vi "AudioTest.SoundCheck Data Log Analysis_Module.vi"(6 "PlotColors":u32[](array[colorbox])=[56063, 16776722, 16730898, 16711925, 6618880], 7 "LimColors":u32[](array[colorbox])=[16448250, 16448250, 16448250, 16448250, 16448250, 16448250], 11 "Module Config":T3={"Name"="AudioGraphs", "Parent Q"=refnum, "Is Child?"=FALSE, "Index"=0, "Dirs"={"Root"=path "", "Config"=path "C:/MTE/Audio Test/Config", "Logs"=path "", "Reports"=path "", "App Data"=path ""}, "Simulate"=FALSE, "SimCtrl"=refnum}) -> ()   [LabVIEW 2018]
uses:
  <vilib>/KATE/Module/Module Config.ctl
  <vilib>/KATE/Queues/Q.Element.ctl
  <vilib>/KATE/Module/Module.Working Dirs.ctl
  Common/Utils/Results/Result.Measurement Item.ctl
  Common/Utils/Results/Result.Measurement and Attribute Item Status.ctl
  TypeDefs/AudioTest.Analysis Data Record.ctl
  Common/Utils/Errors/Error.Error Code List.ctl
  <vilib>/KATE/Queues/Queue Utils.lvlib
  <vilib>/KATE/Files/File Utils.lvlib
  <vilib>/KATE/Time/Time Utils.lvlib
  <vilib>/KATE/Module/Module Utils.lvlib
panel:
  in  "Main Tab":enum32{"Graphs", "Results", "Setup"}(tab)
  in  "Graph - Open Composite":bool
  in  "Go To Results":bool
  in  "Graph Wins - Reset Pos":bool
  in  "Graph Wins - Close":bool
  in  "Graph Wins - Open":bool
  in  "Save to CSV":bool
  in  "X Scale":enum16{"Log", "Linear"}(ring)
  out "Y Units":string
  out "X Units":string
  in  "Next":bool
  in  "Prev":bool
  out "XY Graph":cluster{"X":dbl[], "Y":dbl[]}[](graph)
  in  "Plot":u16(ring)
  in  "SoundCheck Data File":path caption="Data File"
  in  "Load File":bool
  in  "Go To Setup":bool
  in  "Go To Graphs":bool
  out "Meas Data":T1[](array[typedef]) {"Status" items=["LOG", "PASS", "FAIL", "ERROR"]}
  in  "Reinit Config":bool
  out "Graph Cnt":i32
  out "Error":errorcluster
  out "Q Name":string="AudioGraphs"
  in  "Go To Graphs 2":bool
  # "Indiv Graphs"
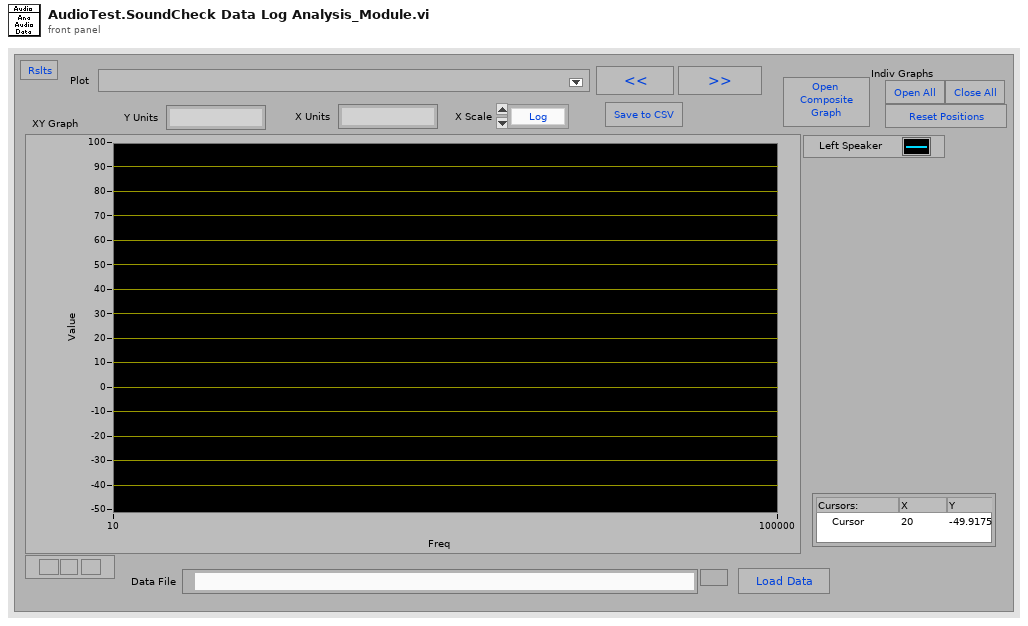
[diagram p1: front panel]
types:
  T1 = typedef "Result.Measurement Item.ctl" = cluster{"Cnt":i32, "Step":string, "Category":string, "Name":string, "Value":string, "Units":string, "LimType":string, "LL":string, "UL":string, "Status":T2, "Code":i32, "Desc":string, "Time":timestamp}
  T2 = typedef "Result.Measurement and Attribute Item Status.ctl" = i32
  T3 = typedef "KATE_Lib.lvlib/Module Utils.lvlib/Module Config.ctl" = cluster{"Name":string, "Parent Q":refnum<queue>, "Is Child?":bool, "Index":i32, "Dirs":T4, "Simulate":bool, "SimCtrl":refnum<vi>}
  T4 = typedef "KATE_Lib.lvlib/Module Utils.lvlib/Module.Working Dirs.ctl" = cluster{"Root":path, "Config":path, "Logs":path, "Reports":path, "App Data":path}
  T5 = typedef "AudioTest.Analysis Data Record.ctl" = cluster{"Name":string, "X Units":string, "Y Units":string, "DataPlots":cluster{"X":dbl[], "Y":dbl[]}[], "LimitPlots":cluster{"X":dbl[], "Y":dbl[]}[], "DataPlotNames":string[], "LimitPlotNames":string[], "Fail":bool}
  T6 = enum32{"invalid app kind", "Development System", "Run Time System", "Student Edition", "Embedded LabVIEW", "Evaluation", "Custom"}
  T7 = cluster{"Graphs":T5[], "Config Dir":path, "PlotColors":u32[], "LimColors":u32[], "PlotWins":cluster{"Name":string, "vi ref":refnum<vi>}[], "PlotComp":cluster{"Name":string, "vi ref":refnum<vi>}}
  T8 = typedef "Error.Error Code List.ctl" = i32
  T9 = typedef "KATE_Lib.lvlib/Queue Utils.lvlib/Q.Element.ctl" = cluster{"Cmd":string, "Sub":string, "Data1":variant, "Data2":variant}
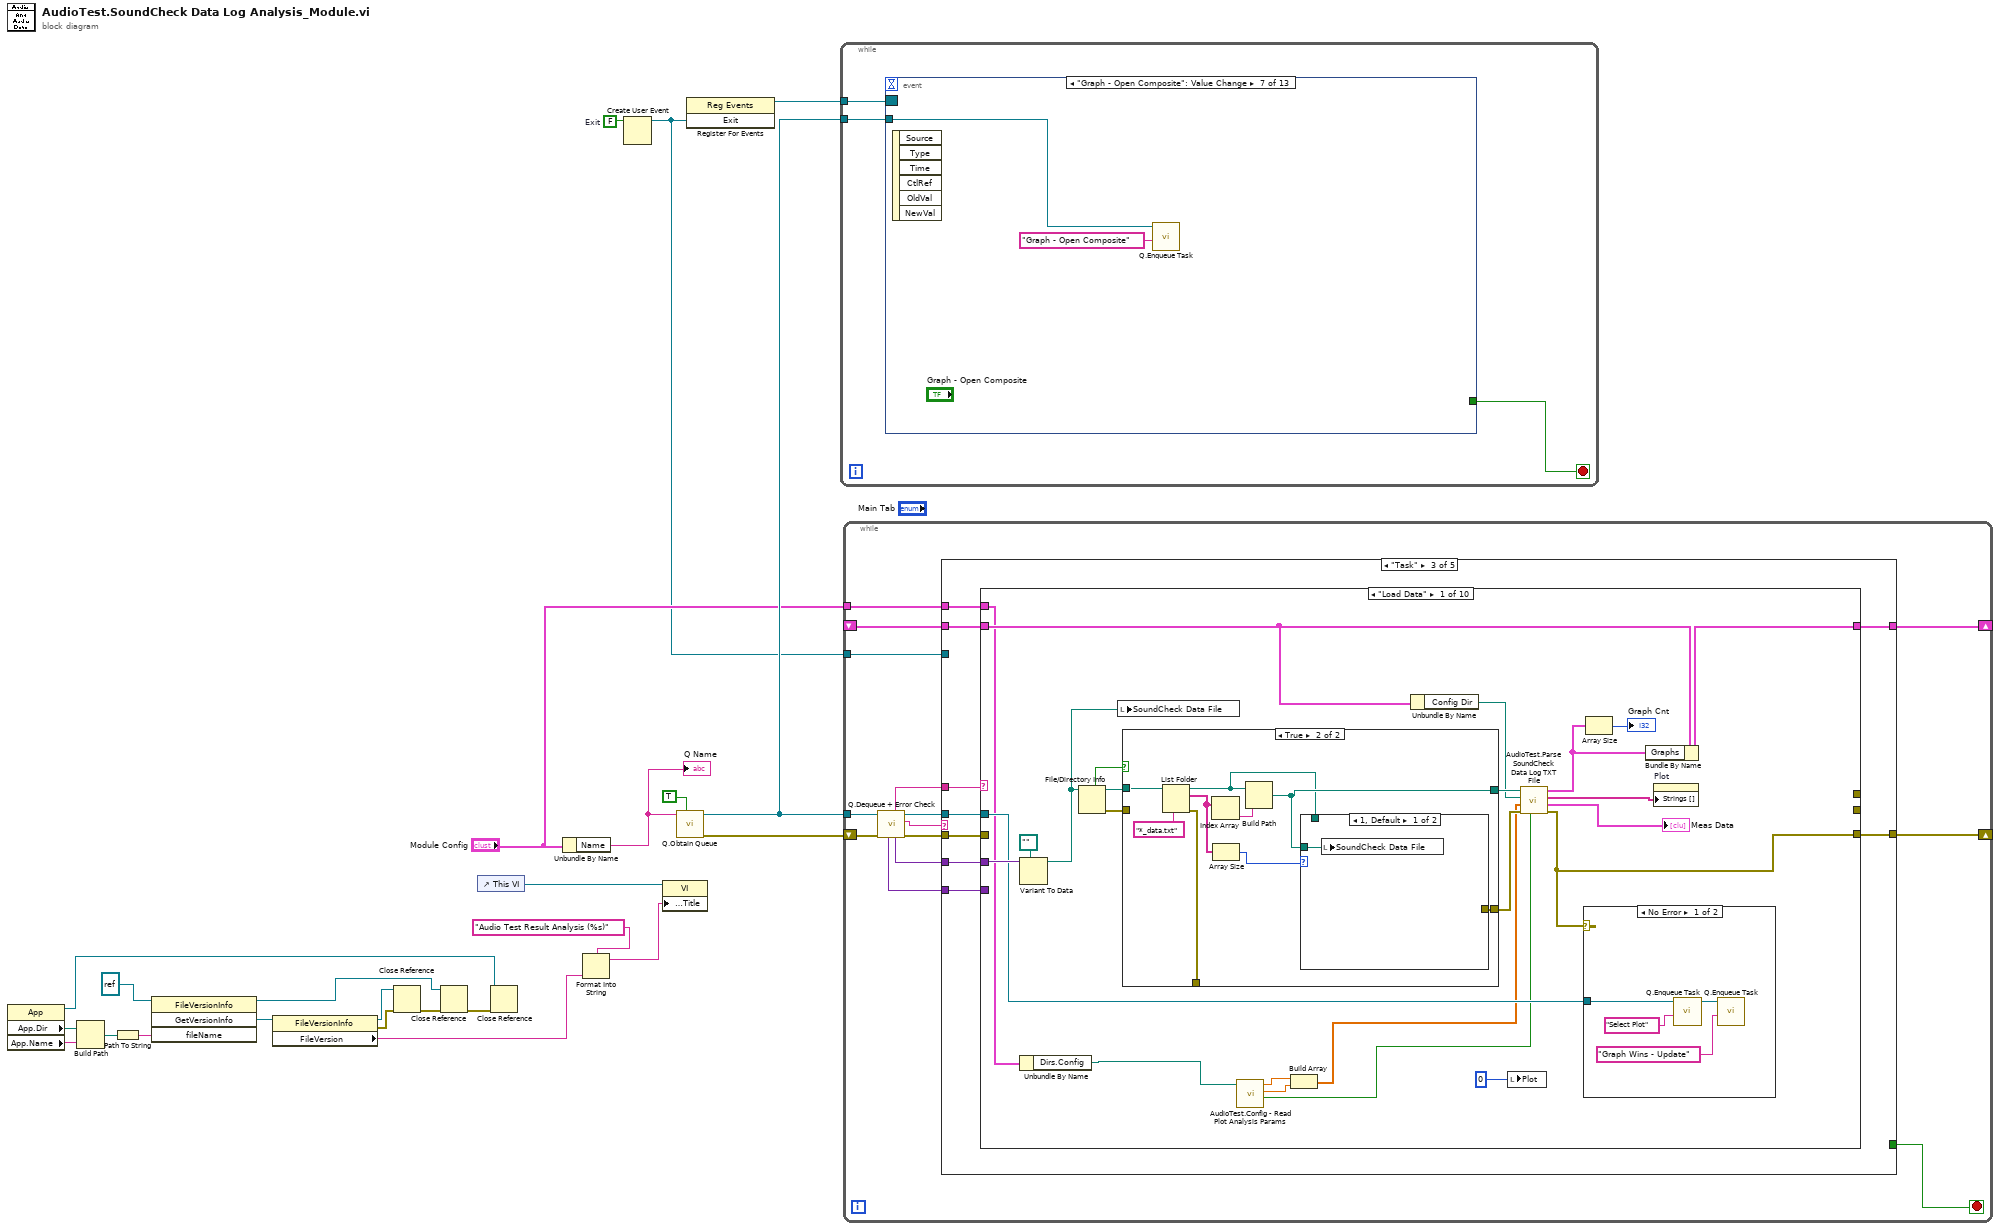
[diagram p0: block diagram]
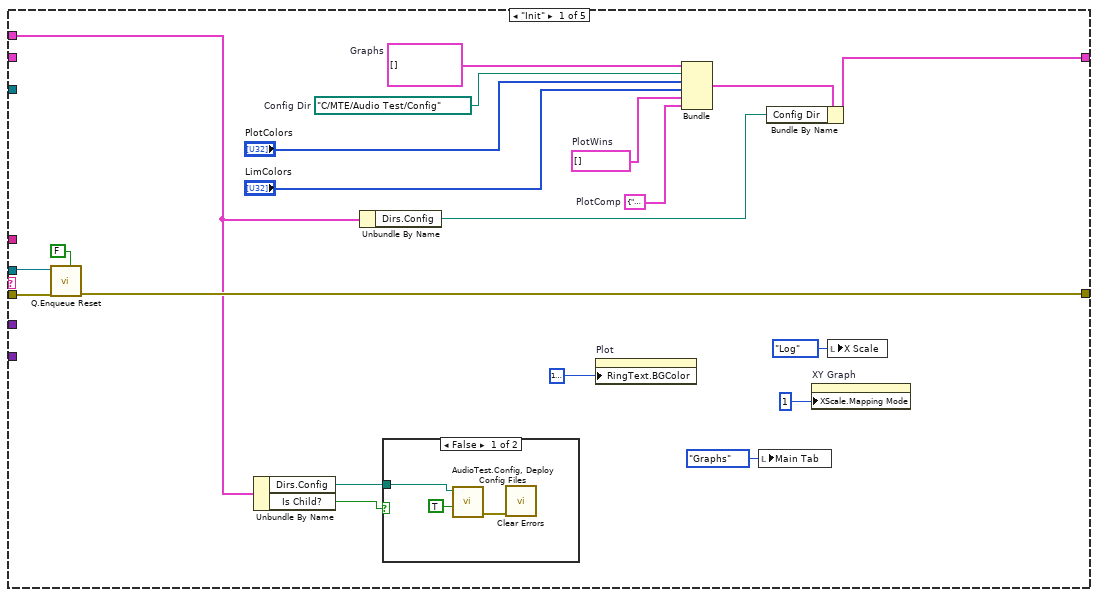
[diagram p2: hidden frame]
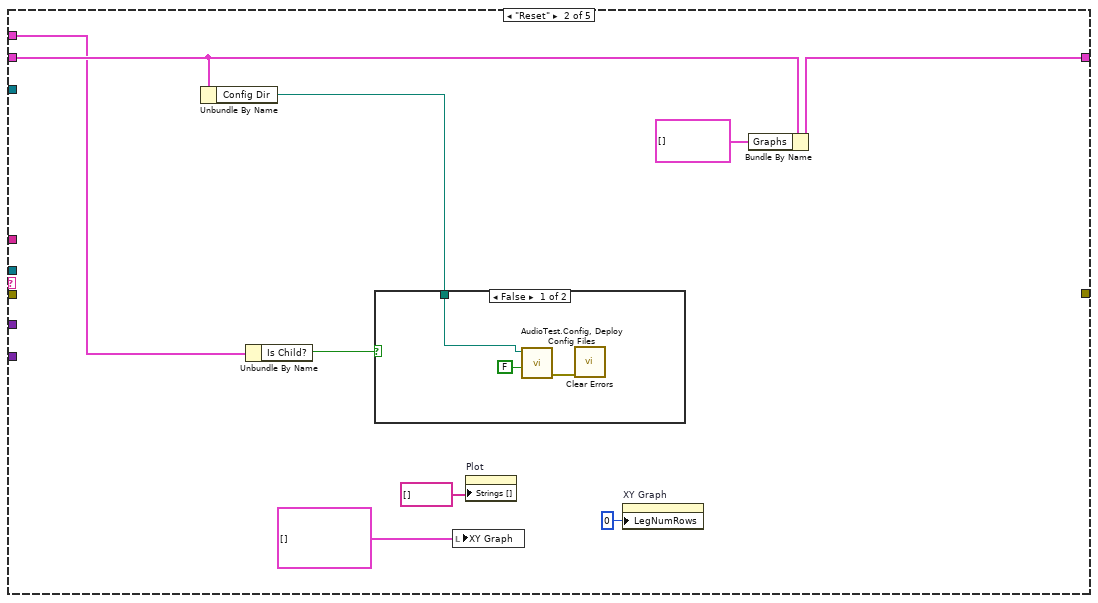
[diagram p4: hidden frame]
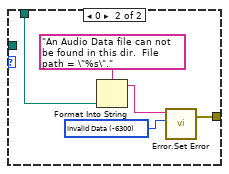
[diagram p8: hidden frame]
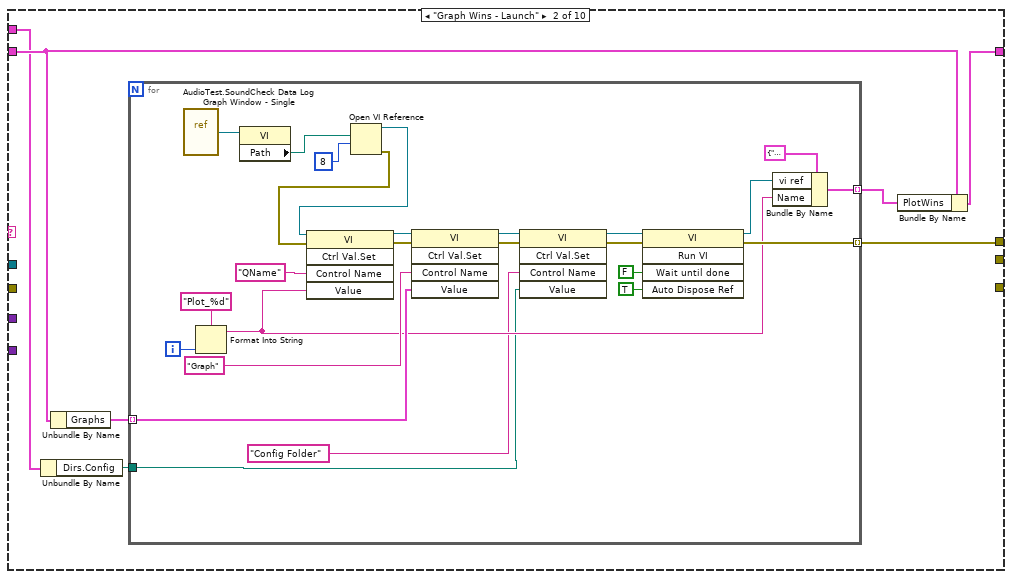
[diagram p9: hidden frame]
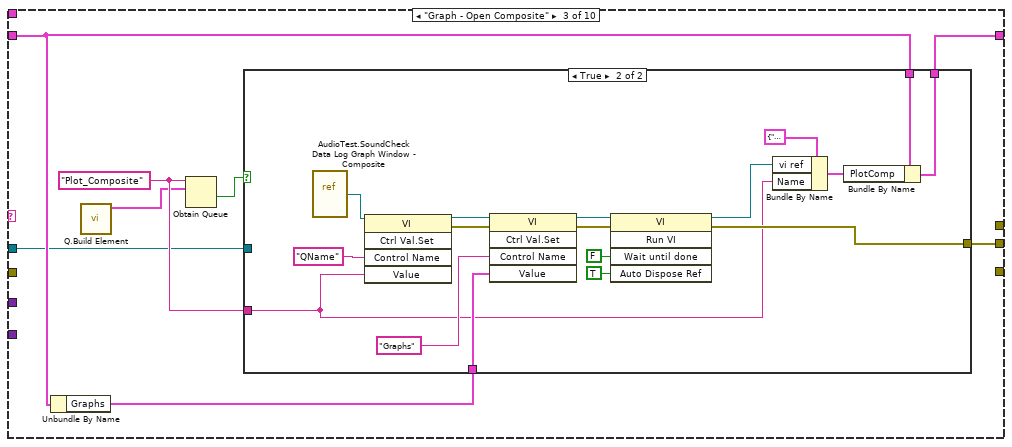
[diagram p10: hidden frame]
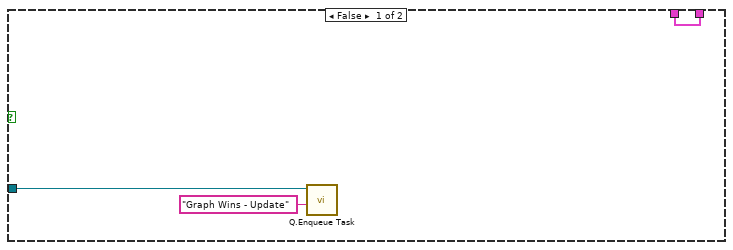
[diagram p11: hidden frame]
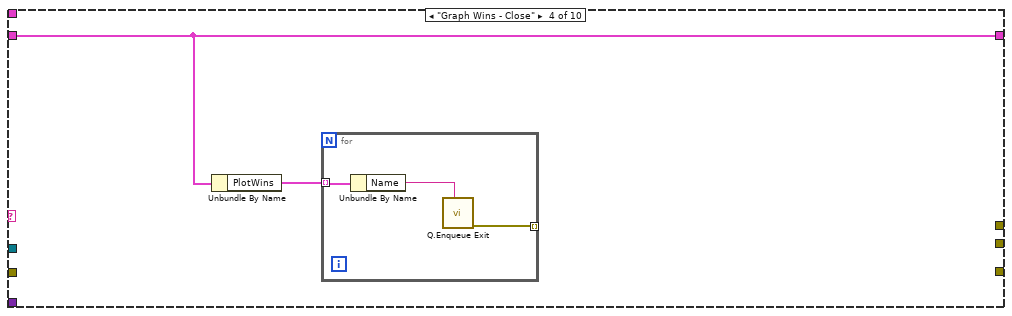
[diagram p12: hidden frame]
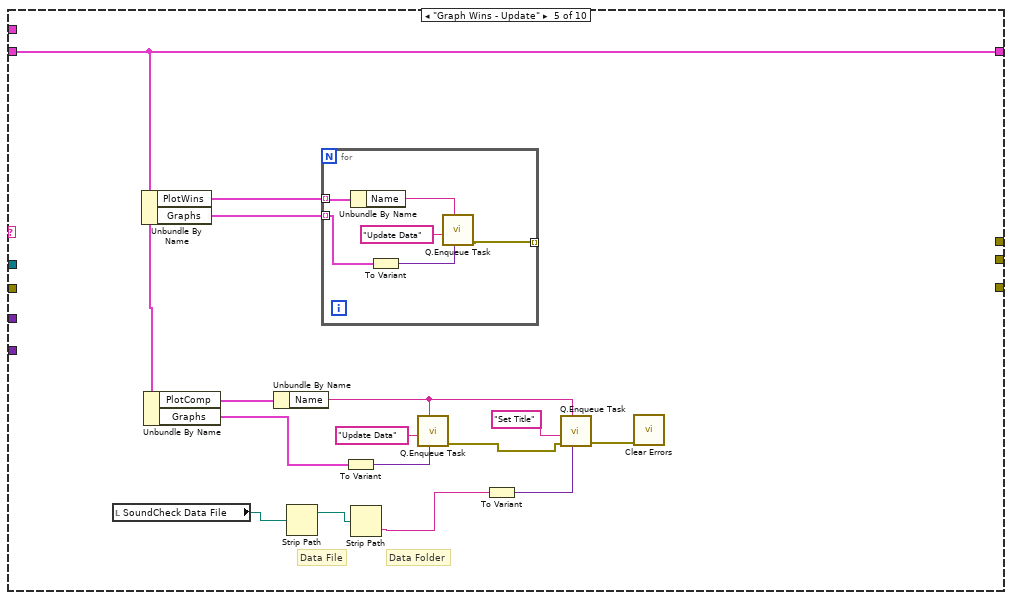
[diagram p13: hidden frame]
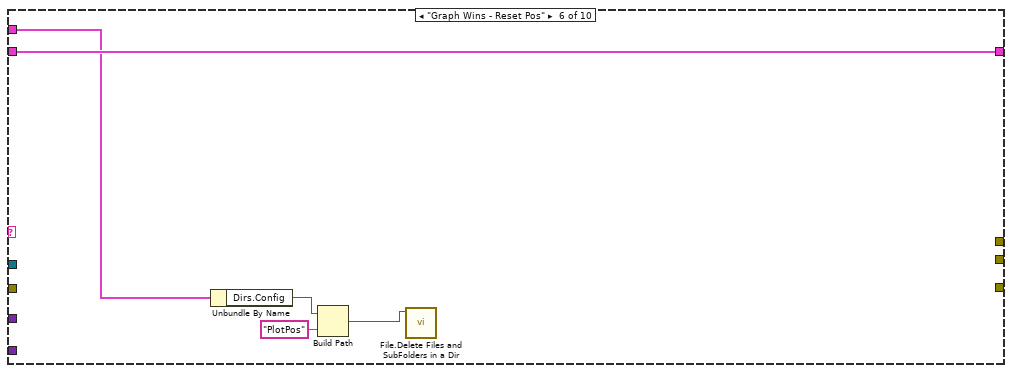
[diagram p14: hidden frame]
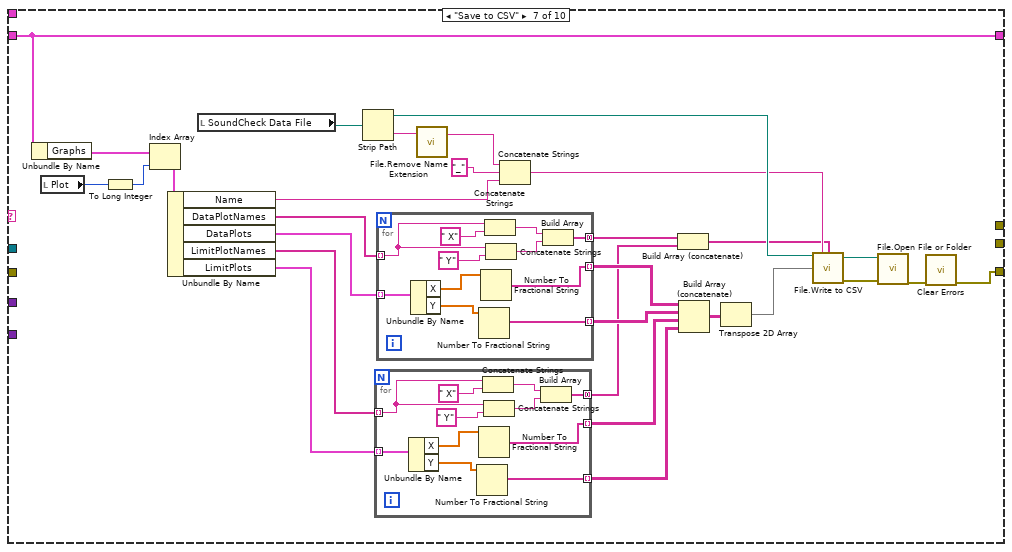
[diagram p15: hidden frame]
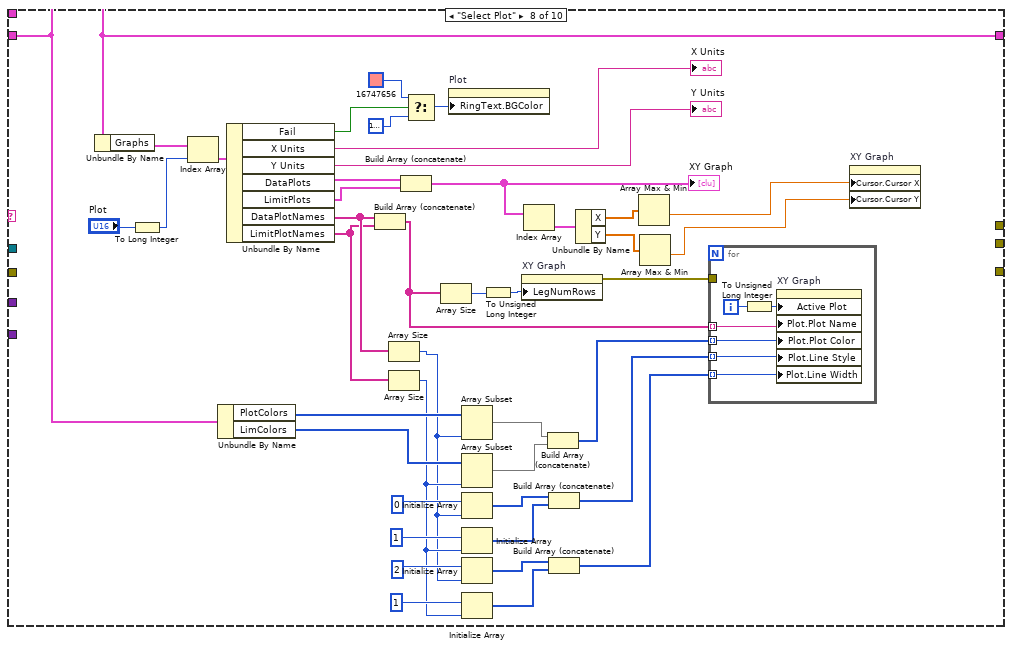
[diagram p16: hidden frame]
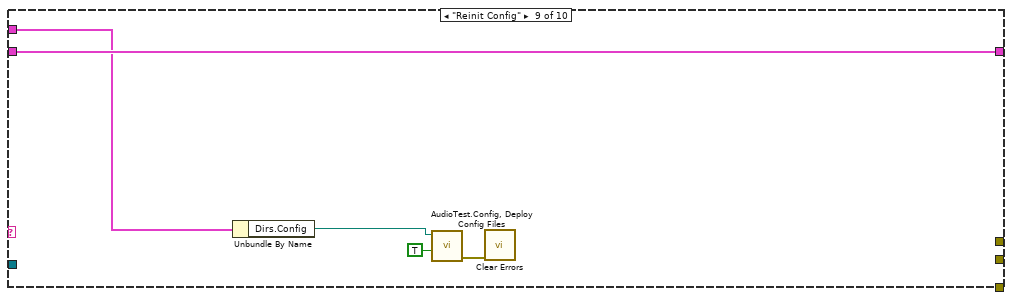
[diagram p17: hidden frame]
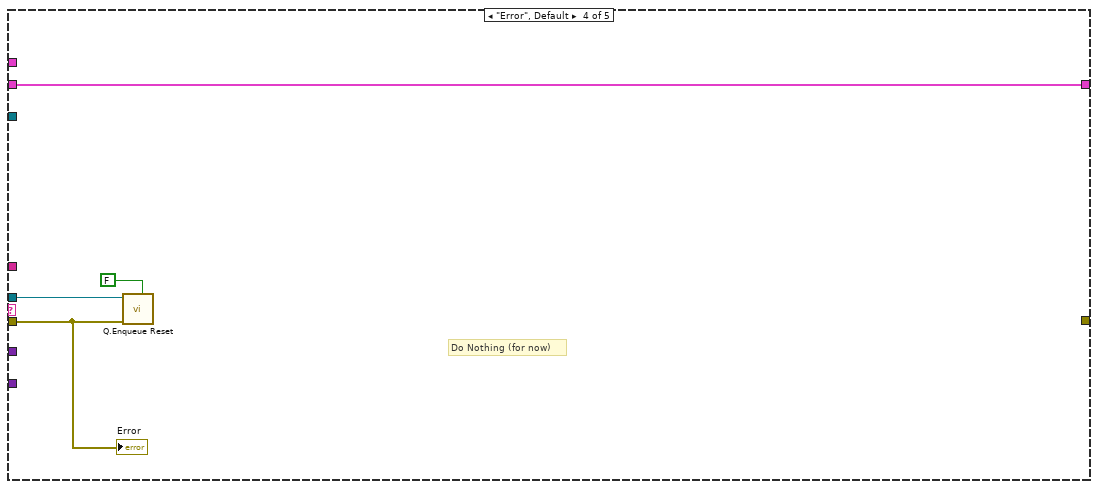
[diagram p19: hidden frame]
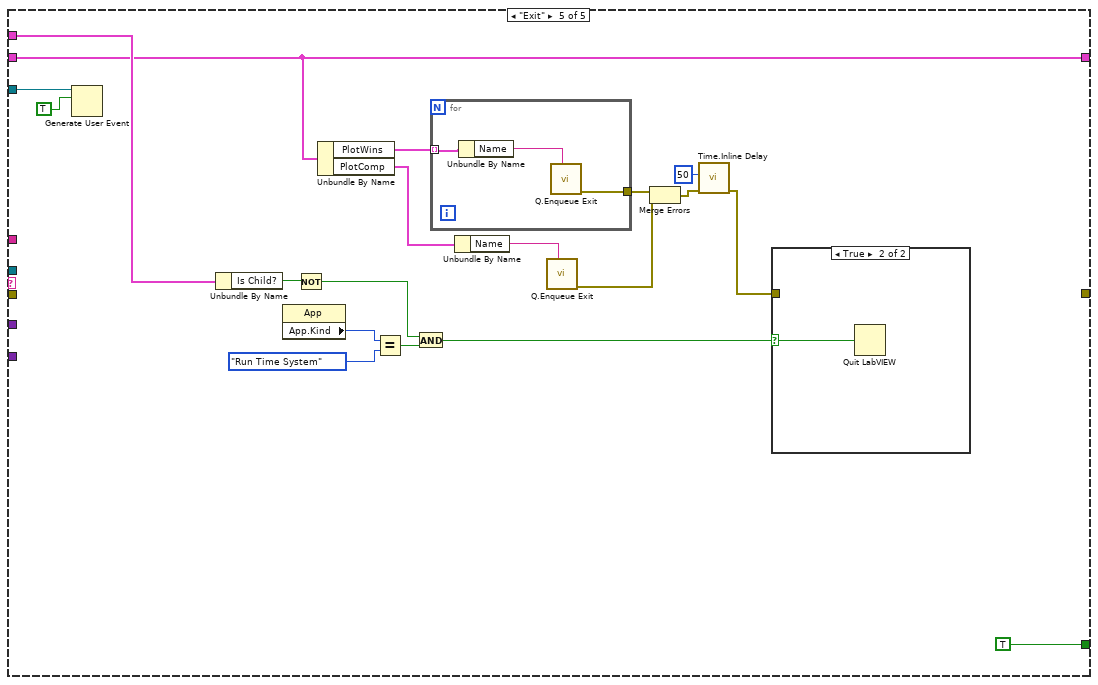
[diagram p20: hidden frame]
diagram:
  w24 = FALSE  # Exit
  n1 = property class="App"() -> (reference out=w3:refnum<vi>, "App.Dir"=w7:path, "App.Name"=w6:string)  [unwired: 2 in, 1 out]
  n2 = Build Path(base path=w7, name or relative path=w6) -> (appended path=w5:path)
  n3 = Path To String(path=w5) -> (string=w13:string)
  n4 = invoke class="FileVersionInfo" method="GetVersionInfo"(reference=refnum<k24> refnum, "fileName"=w13) -> (reference out=w9:refnum<k24>, "GetVersionInfo"=w14:refnum<k24>)  [unwired: 2 in, 2 out]
  n5 = property class="FileVersionInfo"(reference=w14) -> (reference out=w12:refnum<k24>, error out=w11:errorcluster, "FileVersion"=w2:string)  [unwired: 1 in]
  n6 = Close Reference(reference=w12, error in (no error)=w11) -> (error out=w10:errorcluster)
  n7 = Close Reference(reference=w9, error in (no error)=w10) -> (error out=w4:errorcluster)
  n8 = control-ref of="This VI"() -> (w17:refnum<vi>)
  n9 = Close Reference(reference=w3, error in (no error)=w4) -> ()  [unwired: 1 out]
  n10 = Unbundle By Name("Module Config") -> ("Name"=w19:string)
  "Q Name" <- w19
  n11 = Format Into String(format string="Audio Test Result Analysis (%s)", w2) -> (resulting string=w15:string)  [unwired: 2 in, 1 out]
  n12 = Create User Event(user event datatype=w24) -> (user event=w1:refnum<user-event>)  [unwired: 1 in, 1 out]
  n13 = property class="VI"(reference=w17, "Front Panel.Title"=w15) -> ()  [unwired: 1 in, 2 out]
  n14 = call <vilib>:"Q.Obtain Queue.vi"("Enqueue Init"=TRUE, "Q Name"=w19) -> ("error out"=w21:errorcluster, "Q Out"=w20:refnum<queue>)  [unwired: 7 in, 1 out]
  n15 = register-events(w1) -> (reference out=w23:refnum<event-registration>)  [unwired: 2 in, 1 out]
  n16 = while {
    tunnel: w23 -> [w27]
    tunnel: w20 -> [w26]
    stop <- w25 stop-if-true
    n17 = event shown="[6] \"Graph - Open Composite\": Value Change" {
      selector: w27 -> [_ _ _ _ _ _ _ _ _ _ _ _ _]
      dyn-events: _ -> [_ _ _ _ _ _ _ _ _ _ _ _ _]
      timeout: _ -> [_ _ _ _ _ _ _ _ _ _ _ _ _]
      tunnel: w26 -> [w30 _ w42 w44 w46 w49 w53 w54 w56 _ w69 w83 w86]
      tunnel: [_ _ _ _ _ _ _ _ _ _ _ w84 TRUE] -> w25
      event "Load File", "SoundCheck Data File": Value Change {
        n18 = event-data() -> ()  [unwired: 1 in, 6 out]
        n19 = To Variant(anything="SoundCheck Data File") -> (Variant=w28:variant)
        n20 = call <vilib>:"Q.Enqueue Task.vi"("Data1"=w28, "Task Name"="Load Data", "Q In"=w30) -> ()  [unwired: 7 in, 2 out]
      }
      event "Go To Setup", "Go To Results", "Go To Graphs 2", "Go To Graphs": Value Change {
        n21 = event-data() -> ()  [unwired: 1 in, 6 out]
        n22 = Or(x="Go To Graphs 2", y="Go To Graphs") -> (x .or. y?=w33:bool)
        n23 = case shown="False" w33 {
          tunnel: [w38 enum32{"Graphs", "Results", "Setup"}."Graphs" ("Main Tab")] -> w36
          tunnel: "Go To Results" -> [w37 _]
          frame False {
            n24 = case shown="False" w37 {
              tunnel: [enum32{"Graphs", "Results", "Setup"}."Setup" ("Main Tab") enum32{"Graphs", "Results", "Setup"}."Results" ("Main Tab")] -> w38
              frame False {
              }
              frame True {
              }
            }
          }
          frame True {
          }
        }
        n25 = local write "Main Tab"(w36) -> ()
      }
      event "Reinit Config": Value Change {
        n26 = event-data() -> ()  [unwired: 1 in, 6 out]
        n27 = call <vilib>:"Q.Enqueue Task.vi"("Task Name"="Reinit Config", "Q In"=w42) -> ()  [unwired: 8 in, 2 out]
      }
      event "Plot": Value Change {
        n28 = event-data() -> ()  [unwired: 1 in, 6 out]
        n29 = call <vilib>:"Q.Enqueue Task.vi"("Task Name"="Select Plot", "Q In"=w44) -> ()  [unwired: 8 in, 2 out]
      }
      event "Save to CSV": Value Change {
        n30 = event-data() -> ()  [unwired: 1 in, 6 out]
        n31 = call <vilib>:"Q.Enqueue Task.vi"("Task Name"="Save to CSV", "Q In"=w46) -> ()  [unwired: 8 in, 2 out]
      }
      event "Graph Wins - Open": Value Change {
        n32 = event-data() -> ()  [unwired: 1 in, 6 out]
        n33 = call <vilib>:"Q.Enqueue Task.vi"("Task Name"="Graph Wins - Close", "Q In"=w49) -> ("Q Out"=w48:refnum<queue>)  [unwired: 8 in, 1 out]
        n34 = call <vilib>:"Q.Enqueue Task.vi"("Task Name"="Graph Wins - Launch", "Q In"=w48) -> ()  [unwired: 8 in, 2 out]
      }
      event "Graph - Open Composite": Value Change {
        n35 = event-data() -> ()  [unwired: 1 in, 6 out]
        n36 = call <vilib>:"Q.Enqueue Task.vi"("Task Name"="Graph - Open Composite", "Q In"=w53) -> ()  [unwired: 8 in, 2 out]
      }
      event "Graph Wins - Reset Pos": Value Change {
        n37 = event-data() -> ()  [unwired: 1 in, 6 out]
        n38 = call <vilib>:"Q.Enqueue Task.vi"("Task Name"="Graph Wins - Reset Pos", "Q In"=w54) -> ()  [unwired: 8 in, 2 out]
      }
      event "Graph Wins - Close": Value Change {
        n39 = event-data() -> ()  [unwired: 1 in, 6 out]
        n40 = call <vilib>:"Q.Enqueue Task.vi"("Task Name"="Graph Wins - Close", "Q In"=w56) -> ()  [unwired: 8 in, 2 out]
      }
      event "X Scale": Value Change {
        n41 = event-data() -> ()  [unwired: 1 in, 6 out]
        n42 = case shown="\"Log\", Default" "X Scale" {
          tunnel: [u8 1 u8 0] -> w58
          frame "Log", Default {
          }
          frame "Linear" {
          }
        }
        n43 = property on="XY Graph" class="XYGraph (strict)"("XScale.Mapping Mode"=w58) -> ()  [unwired: 2 in, 2 out]
      }
      event "Next", "Prev": Value Change {
        n44 = event-data() -> ()  [unwired: 1 in, 6 out]
        n45 = local read "Graph Cnt"() -> (w65:i32)
        n46 = local read "Plot"() -> (w67:u16)
        n47 = Decrement(x=w65) -> (x-1=w64:i32)
        n48 = To Long Integer(number=w67) -> (32bit integer=w66:i32)
        n49 = case shown="False" "Next" {
          tunnel: w66 -> [w75 w81]
          tunnel: [w71 w79] -> w63
          tunnel: w64 -> [w74 w80]
          frame False {
            n50 = Decrement(x=w75) -> (x-1=w72:i32)
            n51 = Less Than 0?(x=w72) -> (x < 0?=w73:bool)
            n52 = Select(t=w74, s=w73, f=w72) -> (s? t:f=w71:i32)
          }
          frame True {
            n53 = Increment(x=w81) -> (x+1=w76:i32)
            n54 = Greater?(x=w76, y=w80) -> (0:w78:bool)
            n55 = Select(t=0, s=w78, f=w76) -> (s? t:f=w79:i32)
          }
        }
        n56 = To Unsigned Word Integer(number=w63) -> (unsigned 16bit integer=w62:u16)
        n57 = call <vilib>:"Q.Enqueue Task.vi"("Task Name"="Select Plot", "Q In"=w69) -> ()  [unwired: 8 in, 2 out]
        n58 = local write "Plot"(w62) -> ()
      }
      event Panel Close? {
        w84 = TRUE
        n59 = event-data() -> ()  [unwired: 1 in, 4 out]
        n60 = call <vilib>:"Q.Enqueue Exit.vi"("Q In"=w83) -> ("error out"=w82:errorcluster)  [unwired: 9 in, 1 out]
        n61 = call <vilib>:"Clear Errors.vi"("error in (no error)"=w82) -> ()  [unwired: 5 in, 2 out]
        n62 = event-data("Discard?"=w84) -> ()  [unwired: 1 in, 1 out]
      }
      event User Event {
        n63 = event-data() -> ()  [unwired: 1 in, 5 out]
        n64 = call <vilib>:"Q.Enqueue Exit.vi"("Q In"=w86) -> ("error out"=w85:errorcluster)  [unwired: 9 in, 1 out]
        n65 = call <vilib>:"Clear Errors.vi"("error in (no error)"=w85) -> ()  [unwired: 5 in, 2 out]
      }
    }
  }
  n66 = while {
    shift-right: [w93] -> _
    shift-left: w21 -> [w98]
    tunnel: w20 -> [w96]
    shift-right: [w91] -> _
    shift-left: _ -> [w90]
    tunnel: "Module Config" -> [w89]
    tunnel: w1 -> [w88]
    stop <- w92 stop-if-true
    n67 = call <vilib>:"Q.Dequeue + Error Check.vi"("Error In"=w98, "Q In"=w96) -> ("error out"=w99:errorcluster, "Cmd"=w101:string, "Q Out"=w100:refnum<queue>, "Data1"=w95:variant, "Sub"=w97:string, "Data2"=w94:variant)  [unwired: 4 in]
    n68 = case shown="\"Task\"" w101 {
      tunnel: w100 -> [w121 _ w144 w387 _]
      tunnel: w99 -> [w120 _ w143 w386 _]
      tunnel: w97 -> [_ _ w145 _ _]
      tunnel: w95 -> [_ _ w142 _ _]
      tunnel: w94 -> [_ _ w141 _ _]
      tunnel: [w118 _ w138 _ _] -> w93
      tunnel: [_ _ _ _ TRUE] -> w92
      tunnel: [w110 w132 w139 w389 w399] -> w91
      tunnel: w90 -> [_ w131 w140 w389 w399]
      tunnel: w89 -> [w103 w129 w137 _ w403]
      tunnel: w88 -> [_ _ _ _ w391]
      frame "Init" {
        w106 = cluster{"Name":string, "vi ref":refnum<vi>} {"Name"="", "vi ref"=refnum}  # PlotComp
        w108 = cluster{"Name":string, "vi ref":refnum<vi>}[] []  # PlotWins
        w114 = path "C:/MTE/Audio Test/Config"  # Config Dir
        w117 = T5[] []  # Graphs
        n69 = call <vilib>:"Q.Enqueue Reset.vi"("Top of Q(T)"=FALSE, "Error In"=w120, "Q In"=w121) -> ("error out"=w118:errorcluster)  [unwired: 7 in, 1 out]
        n70 = Unbundle By Name(w103) -> ("Dirs.Config"=w104:path, "Is Child?"=w102:bool)
        n71 = Unbundle By Name(w103) -> ("Dirs.Config"=w109:path)
        n72 = case shown="False" w102 {
          tunnel: w104 -> [w123 _]
          frame False {
            n73 = call "AudioTest.Config, Deploy Config Files.vi"("SkipIfExists(F)/Overwrite(T)"=TRUE, "Config Folder"=w123) -> ("error out"=w124:errorcluster)  [unwired: 9 in]
            n74 = call <vilib>:"Clear Errors.vi"("error in (no error)"=w124) -> ()  [unwired: 5 in, 2 out]
          }
          frame True {
          }
        }
        n75 = property on="Plot" class="Ring (strict)"("RingText.BGColor"=u32 16777216 ("Color Box")) -> ()  [unwired: 2 in, 2 out]
        n76 = Bundle("Graphs"=w117, "Config Dir"=w114, "PlotColors"="PlotColors", "LimColors"="LimColors", "PlotWins"=w108, "PlotComp"=w106) -> (w111:T7)  [unwired: 1 in]
        n77 = local write "Main Tab"(enum32{"Graphs", "Results", "Setup"}."Graphs" ("Main Tab")) -> ()
        n78 = Bundle By Name(cluster=w111, "Config Dir"=w109) -> (w110:T7)
        n79 = property on="XY Graph" class="XYGraph (strict)"("XScale.Mapping Mode"=u8 1) -> ()  [unwired: 2 in, 2 out]
        n80 = local write "X Scale"(enum16{"Log", "Linear"}."Log" ("X Scale")) -> ()
      }
      frame "Reset" {
        n81 = Unbundle By Name(w131) -> ("Config Dir"=w130:path)
        n82 = Unbundle By Name(w129) -> ("Is Child?"=w128:bool)
        n83 = case shown="False" w128 {
          tunnel: w130 -> [w134 _]
          frame False {
            n84 = call "AudioTest.Config, Deploy Config Files.vi"("SkipIfExists(F)/Overwrite(T)"=FALSE, "Config Folder"=w134) -> ("error out"=w135:errorcluster)  [unwired: 9 in]
            n85 = call <vilib>:"Clear Errors.vi"("error in (no error)"=w135) -> ()  [unwired: 5 in, 2 out]
          }
          frame True {
          }
        }
        n86 = local write "XY Graph"(cluster{"X":dbl[], "Y":dbl[]}[] [] ("appended array")) -> ()
        n87 = property on="Plot" class="Ring (strict)"("Strings []"=string[] []) -> ()  [unwired: 2 in, 2 out]
        n88 = property on="XY Graph" class="XYGraph (strict)"("LegNumRows"=u32 0 ("Legend:Number of Rows")) -> ()  [unwired: 2 in, 2 out]
        n89 = Bundle By Name(cluster=w131, "Graphs"=T5[] []) -> (w132:T7)
      }
      frame "Task" {
        n90 = case shown="\"Load Data\"" w145 {
          tunnel: w144 -> [w160 _ w223 _ _ _ _ _ _ _]
          tunnel: w143 -> [_ _ _ _ _ _ _ _ _ _]
          tunnel: w142 -> [w163 _ _ _ _ _ _ _ _ _]
          tunnel: w141 -> [_ _ _ _ _ _ _ _ _ _]
          tunnel: w140 -> [w156 w195 w225 w251 w267 w280 w305 w361 w384 w385]
          tunnel: [w161 w194 w224 w251 w267 w280 w305 w361 w384 w385] -> w139
          tunnel: [w159 _ _ _ _ _ w282 _ _ _] -> w138
          tunnel: [_ w192 _ _ _ _ _ _ _ _] -> _
          tunnel: w137 -> [w149 w191 _ _ _ w279 _ _ w382 _]
          tunnel: [_ _ w228 _ _ _ _ _ _ _] -> _
          frame "Load Data" {
            n91 = Unbundle By Name(w149) -> ("Dirs.Config"=w148:path)
            n92 = Variant To Data(type=path "", Variant=w163) -> (data=w158:path)  [unwired: 1 in, 1 out]
            n93 = File/Directory Info(path=w158) -> (path out=w165:path, directory=w166:bool, error out=w168:errorcluster)  [unwired: 1 in, 4 out]
            n94 = local write "SoundCheck Data File"(w158) -> ()
            n95 = case shown="True" w166 {
              tunnel: w165 -> [w174 w183]
              tunnel: [w174 w181] -> w167
              tunnel: w168 -> [_ _]
              tunnel: [_ w180] -> _
              tunnel: [_ w176] -> w169
              frame False {
              }
              frame True {
                n96 = List Folder(path=w183, pattern="*_data.txt") -> (path out=w175:path, filenames=w179:string[], error out=w180:errorcluster)  [unwired: 2 in, 1 out]
                n97 = Index Array(array=w179) -> (element=w177:string)  [unwired: 1 in]
                n98 = Array Size(array=w179) -> (size(s)=w178:i32)
                n99 = Build Path(base path=w175, name or relative path=w177) -> (appended path=w181:path)
                n100 = case shown="1, Default" w178 {
                  tunnel: w181 -> [w184 _]
                  tunnel: [_ w186] -> w176
                  tunnel: w175 -> [_ w185]
                  frame 1, Default {
                    n101 = local write "SoundCheck Data File"(w184) -> ()
                  }
                  frame 0 {
                    w187 = T8 -6300 items=["No Error"=0, "Abort"=-2, "Misc"=-5000, "Fixture Error"=-5100, "File IO - General"=-5200, "FIle IO - Config Error"=-5201, "Instrument - General"=-5300, "Instrument - Serial Com"=-5301, "Instrument - Camera"=-5302, "Instrument - PS"=-5303, "Instrument - Oscilloscope"=-5304, "Instrument - Function Gen"=-5305, "Instrument - Load"=-5306, "Instrument - Meter"=-5307, "Instrument - Power Control"=-5308, "Instrument - Motion"=-5309, "Instrument - RF"=-5310, "System Exe"=-5400, "Image Processing"=-5500, "Communication"=-5600, "Script - Syntax Error"=-6000, "Script - Invalid Name or Param"=-6100, "Script - Timeout"=-6200, "Invalid Data"=-6300, "FW Update Error"=-6500] ("Std Code")
                    n102 = Format Into String(format string="An Audio Data file can not be found in this dir.  File path = \"%s\"." ("Desc"), w185) -> (resulting string=w189:string)  [unwired: 2 in, 1 out]
                    n103 = call "Error.Set Error.vi"("Code"=w187, "Desc"=w189) -> ("error out"=w186:errorcluster)  [unwired: 5 in]
                  }
                }
              }
            }
            n104 = call "AudioTest.Config - Read Plot Analysis Params.vi"("Config Dir"=w148) -> ("Avg(F)/Float(T)"=w146:bool, "End Freq"=w150:dbl, "Start Freq"=w151:dbl)  [unwired: 8 in]
            n105 = Build Array(w151, w150) -> (w147:dbl[])
            n106 = Unbundle By Name(w156) -> ("Config Dir"=w155:path)
            n107 = local write "Plot"(0) -> ()
            n108 = call "AudioTest.Parse SoundCheck Data Log TXT File.vi"("Lim Center at Average(f), Float at center"=w146, "error in"=w169, "Start_End"=w147, "Config Folder"=w155, "SoundCheck Data File"=w167) -> ("error out"=w159:errorcluster, "Meas Rslt"=→"Meas Data":T1[], "Graph Names"=w157:string[], "Graphs"=w154:T5[])  [unwired: 3 in]
            n109 = case shown="No Error" w159 {
              tunnel: w160 -> [w172 _]
              frame No Error {
                n110 = call <vilib>:"Q.Enqueue Task.vi"("Task Name"="Select Plot", "Q In"=w172) -> ("Q Out"=w171:refnum<queue>)  [unwired: 8 in, 1 out]
                n111 = call <vilib>:"Q.Enqueue Task.vi"("Task Name"="Graph Wins - Update", "Q In"=w171) -> ()  [unwired: 8 in, 2 out]
              }
              frame Error {
              }
            }
            n112 = Array Size(array=w154) -> (size(s)=→"Graph Cnt":i32)
            n113 = Bundle By Name(cluster=w156, "Graphs"=w154) -> (w161:T7)
            n114 = property on="Plot" class="Ring (strict)"("Strings []"=w157) -> ()  [unwired: 2 in, 2 out]
          }
          frame "Graph Wins - Launch" {
            n115 = Unbundle By Name(w191) -> ("Dirs.Config"=w190:path)
            n116 = Unbundle By Name(w195) -> ("Graphs"=w196:T5[])
            n117 = for {
              tunnel: w196 -> [w213] mode=indexing
              tunnel: [w212] -> w192 mode=indexing
              tunnel: [w208] -> w193 mode=indexing
              tunnel: w190 -> [w197]
              i -> [w214]
              n118 = vi-ref "AudioTest.SoundCheck Data Log Graph Window - Single.vi"() -> (w207:refnum<vi>)
              n119 = Format Into String(format string="Plot_%d", w214) -> (resulting string=w210:string)  [unwired: 2 in, 1 out]
              n120 = property class="VI"(reference=w207) -> ("Path"=w206:path)  [unwired: 1 in, 2 out]
              n121 = Open VI Reference(vi path=w206, options=8) -> (vi reference=w205:refnum<vi>, error out=w203:errorcluster)  [unwired: 4 in]
              n122 = invoke class="VI" method="Ctrl Val.Set"(reference=w205, error in=w203, "Control Name"="QName", "Value"=w210) -> (reference out=w219:refnum<vi>, error out=w218:errorcluster)  [unwired: 1 in, 3 out]
              n123 = invoke class="VI" method="Ctrl Val.Set"(reference=w219, error in=w218, "Control Name"="Graph", "Value"=w213) -> (reference out=w202:refnum<vi>, error out=w201:errorcluster)  [unwired: 1 in, 3 out]
              n124 = invoke class="VI" method="Ctrl Val.Set"(reference=w202, error in=w201, "Control Name"="Config Folder", "Value"=w197) -> (reference out=w199:refnum<vi>, error out=w200:errorcluster)  [unwired: 1 in, 3 out]
              n125 = invoke class="VI" method="Run VI"(reference=w199, error in=w200, "Wait until done"=FALSE ("Wait Until Done"), "Auto Dispose Ref"=TRUE ("Auto Dispose Reference")) -> (reference out=w209:refnum<vi>, error out=w212:errorcluster)  [unwired: 1 in, 3 out]
              n126 = Bundle By Name(cluster=cluster{"Name":string, "vi ref":refnum<vi>} {"Name"="", "vi ref"=refnum} ("Service"), "vi ref"=w209, "Name"=w210) -> (w208:cluster{"Name":string, "vi ref":refnum<vi>})
            }
            n127 = Bundle By Name(cluster=w195, "PlotWins"=w193) -> (w194:T7)
          }
          frame "Graph - Open Composite" {
            w227 = "Plot_Composite"
            n128 = Unbundle By Name(w225) -> ("Graphs"=w229:T5[])
            n129 = call <vilib>:"Q.Build Element.vi"() -> ("Q.Element"=w222:T9)  [unwired: 11 in]
            n130 = Obtain Queue(name (unnamed)=w227, element data type=w222) -> (created new?=w226:bool)  [unwired: 3 in, 2 out]
            n131 = case shown="True" w226 {
              tunnel: w229 -> [_ w249]
              tunnel: [_ w237] -> w228
              tunnel: w227 -> [_ w236]
              tunnel: w225 -> [w232 w234]
              tunnel: [w232 w233] -> w224
              tunnel: w223 -> [w231 _]
              frame False {
                n132 = call <vilib>:"Q.Enqueue Task.vi"("Task Name"="Graph Wins - Update", "Q In"=w231) -> ()  [unwired: 8 in, 2 out]
              }
              frame True {
                n133 = vi-ref "AudioTest.SoundCheck Data Log Graph Window - Composite.vi"() -> (w238:refnum<vi>)
                n134 = invoke class="VI" method="Ctrl Val.Set"(reference=w238, "Control Name"="QName", "Value"=w236) -> (reference out=w246:refnum<vi>, error out=w245:errorcluster)  [unwired: 2 in, 3 out]
                n135 = invoke class="VI" method="Ctrl Val.Set"(reference=w246, error in=w245, "Control Name"="Graphs", "Value"=w249) -> (reference out=w240:refnum<vi>, error out=w239:errorcluster)  [unwired: 1 in, 3 out]
                n136 = invoke class="VI" method="Run VI"(reference=w240, error in=w239, "Wait until done"=FALSE ("Wait Until Done"), "Auto Dispose Ref"=TRUE ("Auto Dispose Reference")) -> (reference out=w241:refnum<vi>, error out=w237:errorcluster)  [unwired: 1 in, 3 out]
                n137 = Bundle By Name(cluster=cluster{"Name":string, "vi ref":refnum<vi>} {"Name"="", "vi ref"=refnum} ("Service"), "vi ref"=w241, "Name"=w236) -> (w235:cluster{"Name":string, "vi ref":refnum<vi>})
                n138 = Bundle By Name(cluster=w234, "PlotComp"=w235) -> (w233:T7)
              }
            }
          }
          frame "Graph Wins - Close" {
            n139 = Unbundle By Name(w251) -> ("PlotWins"=w250:cluster{"Name":string, "vi ref":refnum<vi>}[])
            n140 = for {
              tunnel: w250 -> [w254] mode=indexing
              tunnel: [w252] -> _ mode=indexing
              n141 = Unbundle By Name(w254) -> ("Name"=w253:string)
              n142 = call <vilib>:"Q.Enqueue Exit.vi"("Q Name"=w253) -> ("error out"=w252:errorcluster)  [unwired: 9 in, 1 out]
            }
          }
          frame "Graph Wins - Update" {
            # "Data Folder"
            # "Data File"
            n143 = local read "SoundCheck Data File"() -> (w258:path)
            n144 = Unbundle By Name(w267) -> ("PlotWins"=w269:cluster{"Name":string, "vi ref":refnum<vi>}[], "Graphs"=w268:T5[])
            n145 = Unbundle By Name(w267) -> ("PlotComp"=w264:cluster{"Name":string, "vi ref":refnum<vi>}, "Graphs"=w263:T5[])
            n146 = Unbundle By Name(w264) -> ("Name"=w260:string)
            n147 = Strip Path(path=w258) -> (stripped path=w257:path)  [unwired: 1 out]
            n148 = for {
              tunnel: w269 -> [w275] mode=indexing
              tunnel: [w271] -> _ mode=indexing
              tunnel: w268 -> [w274] mode=indexing
              n149 = Unbundle By Name(w275) -> ("Name"=w272:string)
              n150 = To Variant(anything=w274) -> (Variant=w273:variant)
              n151 = call <vilib>:"Q.Enqueue Task.vi"("Data1"=w273, "Q Name"=w272, "Task Name"="Update Data") -> ("error out"=w271:errorcluster)  [unwired: 7 in, 1 out]
            }
            n152 = To Variant(anything=w263) -> (Variant=w265:variant)
            n153 = Strip Path(path=w257) -> (name=w256:string)  [unwired: 1 out]
            n154 = call <vilib>:"Q.Enqueue Task.vi"("Data1"=w265, "Q Name"=w260, "Task Name"="Update Data") -> ("error out"=w255:errorcluster)  [unwired: 7 in, 1 out]
            n155 = To Variant(anything=w256) -> (Variant=w262:variant)
            n156 = call <vilib>:"Q.Enqueue Task.vi"("Data1"=w262, "Q Name"=w260, "Error In"=w255, "Task Name"="Set Title") -> ("error out"=w259:errorcluster)  [unwired: 6 in, 1 out]
            n157 = call <vilib>:"Clear Errors.vi"("error in (no error)"=w259) -> ()  [unwired: 5 in, 2 out]
          }
          frame "Graph Wins - Reset Pos" {
            n158 = Unbundle By Name(w279) -> ("Dirs.Config"=w277:path)
            n159 = Build Path(base path=w277, name or relative path="PlotPos") -> (appended path=w276:path)
            n160 = call <vilib>:"File.Delete Files and SubFolders in a Dir.vi"("Dir"=w276) -> ()  [unwired: 9 in, 2 out]
          }
          frame "Save to CSV" {
            n161 = Unbundle By Name(w305) -> ("Graphs"=w309:T5[])
            n162 = local read "Plot"() -> (w308:u16)
            n163 = To Long Integer(number=w308) -> (32bit integer=w307:i32)
            n164 = Index Array(array=w309, index=w307) -> (element=w306:T5)
            n165 = Unbundle By Name(w306) -> ("Name"=w300:string, "DataPlotNames"=w298:string[], "DataPlots"=w299:cluster{"X":dbl[], "Y":dbl[]}[], "LimitPlotNames"=w291:string[], "LimitPlots"=w290:cluster{"X":dbl[], "Y":dbl[]}[])
            n166 = local read "SoundCheck Data File"() -> (w304:path)
            n167 = Strip Path(path=w304) -> (stripped path=w295:path, name=w303:string)
            n168 = for {
              tunnel: w290 -> [w320] mode=indexing
              tunnel: w291 -> [w316] mode=indexing
              tunnel: [w314] -> w289 mode=indexing
              tunnel: [w313] -> w288 mode=indexing
              tunnel: [w310] -> w287 mode=concatenating
              n169 = Unbundle By Name(w320) -> ("X"=w319:dbl[], "Y"=w318:dbl[])
              n170 = Number To Fractional String(number=w318) -> (F-format string=w313:string[])  [unwired: 3 in]
              n171 = Number To Fractional String(number=w319) -> (F-format string=w314:string[])  [unwired: 3 in]
              n172 = Concatenate Strings(w316, " X" ("string")) -> (w312:string)
              n173 = Concatenate Strings(w316, " Y" ("string")) -> (w311:string)
              n174 = Build Array(w312, w311) -> (w310:string[])
            }
            n175 = for {
              tunnel: w299 -> [w331] mode=indexing
              tunnel: w298 -> [w327] mode=indexing
              tunnel: [w325] -> w297 mode=indexing
              tunnel: [w324] -> w296 mode=indexing
              tunnel: [w321] -> w292 mode=concatenating
              n176 = Unbundle By Name(w331) -> ("X"=w330:dbl[], "Y"=w329:dbl[])
              n177 = Number To Fractional String(number=w329) -> (F-format string=w324:string[])  [unwired: 3 in]
              n178 = Number To Fractional String(number=w330) -> (F-format string=w325:string[])  [unwired: 3 in]
              n179 = Concatenate Strings(w327, " X" ("string")) -> (w323:string)
              n180 = Concatenate Strings(w327, " Y" ("string")) -> (w322:string)
              n181 = Build Array(w323, w322) -> (w321:string[])
            }
            n182 = call <vilib>:"File.Remove Name Extension.vi"("File Name"=w303) -> ("Name Less Ext"=w301:string)  [unwired: 1 in, 1 out]
            n183 = Concatenate Strings(w301, "_", w300) -> (w294:string)
            n184 = Build Array (concatenate)(w292, w287) -> (w286:string[])
            n185 = Build Array (concatenate)(w297, w296, w289, w288) -> (w285:string[][])
            n186 = Transpose 2D Array(2D array=w285) -> (transposed array=w293:string[][])
            n187 = call <vilib>:"File.Write to CSV.vi"("Folder"=w295, "FileRootName"=w294, "Header"=w286, "2D"=w293) -> ("File Path"=w284:path, "error out"=w283:errorcluster)  [unwired: 10 in]
            n188 = call <vilib>:"File.Open File or Folder.vi"("Error In"=w283, "Path"=w284) -> ("Error Out"=w281:errorcluster)  [unwired: 9 in]
            n189 = call <vilib>:"Clear Errors.vi"("error in (no error)"=w281) -> ("error out"=w282:errorcluster)  [unwired: 5 in, 1 out]
          }
          frame "Select Plot" {
            n190 = Unbundle By Name(w361) -> ("Graphs"=w368:T5[])
            n191 = To Long Integer(number="Plot") -> (32bit integer=w371:i32)
            n192 = Index Array(array=w368, index=w371) -> (element=w369:T5)
            n193 = Unbundle By Name(w361) -> ("PlotColors"=w358:u32[], "LimColors"=w357:u32[])
            n194 = Unbundle By Name(w369) -> ("Fail"=w338:bool, "X Units"=→"X Units":string, "Y Units"=→"Y Units":string, "DataPlots"=w367:cluster{"X":dbl[], "Y":dbl[]}[], "LimitPlots"=w366:cluster{"X":dbl[], "Y":dbl[]}[], "DataPlotNames"=w360:string[], "LimitPlotNames"=w359:string[])
            n195 = Build Array (concatenate)(w360, w359) -> (w362:string[])
            n196 = Array Size(array=w360) -> (size(s)=w343:i32)
            n197 = Array Size(array=w359) -> (size(s)=w344:i32)
            n198 = Build Array (concatenate)(w367, w366) -> (w337:cluster{"X":dbl[], "Y":dbl[]}[])
            "XY Graph" <- w337
            n199 = Select(t=u32 16747656 ("Color Box"), s=w338, f=u32 16777216 ("Color Box")) -> (s? t:f=w340:u32)
            n200 = Array Size(array=w362) -> (size(s)=w365:i32)
            n201 = property on="Plot" class="Ring (strict)"("RingText.BGColor"=w340) -> ()  [unwired: 2 in, 2 out]
            n202 = Array Subset(array=w358, length=w343) -> (w356:u32[])  [unwired: 1 in]
            n203 = Array Subset(array=w357, length=w344) -> (w355:u32[])  [unwired: 1 in]
            n204 = Initialize Array(u8 0 ("Plot.Line Style"), w343) -> (w351:u8[])
            n205 = Initialize Array(u8 1 ("Plot.Line Style"), w344) -> (w350:u8[])
            n206 = Initialize Array(u8 2 ("Plot.Line Style"), w343) -> (w347:u8[])
            n207 = Initialize Array(u8 1 ("Plot.Line Style"), w344) -> (w348:u8[])
            n208 = To Unsigned Long Integer(number=w365) -> (unsigned 32bit integer=w364:u32)
            n209 = property on="XY Graph" class="XYGraph (strict)"("LegNumRows"=w364) -> (error out=w363:errorcluster)  [unwired: 2 in, 1 out]
            n210 = Index Array(array=w337) -> (element=w336:cluster{"X":dbl[], "Y":dbl[]})  [unwired: 1 in]
            n211 = Build Array (concatenate)(w356, w355) -> (w354:u32[])
            n212 = Build Array (concatenate)(w351, w350) -> (w349:u8[])
            n213 = Build Array (concatenate)(w347, w348) -> (w342:u8[])
            n214 = Unbundle By Name(w336) -> ("X"=w335:dbl[], "Y"=w334:dbl[])
            n215 = Array Max & Min(array=w335) -> (min value=w333:dbl)  [unwired: 3 out]
            n216 = Array Max & Min(array=w334) -> (min value=w332:dbl)  [unwired: 3 out]
            n217 = for {
              tunnel: w362 -> [w377] mode=indexing
              tunnel: w363 -> [_]
              tunnel: w354 -> [w376] mode=indexing
              tunnel: w349 -> [w375] mode=indexing
              tunnel: w342 -> [w374] mode=indexing
              i -> [w378]
              n218 = To Unsigned Long Integer(number=w378) -> (unsigned 32bit integer=w379:u32)
              n219 = property on="XY Graph" class="XYGraph (strict)"("Active Plot"=w379, "Plot.Plot Name"=w377, "Plot.Plot Color"=w376, "Plot.Line Style"=w375, "Plot.Line Width"=w374) -> ()  [unwired: 2 in, 2 out]
            }
            n220 = property on="XY Graph" class="XYGraph (strict)"("Cursor.Cursor X"=w333, "Cursor.Cursor Y"=w332) -> ()  [unwired: 2 in, 2 out]
          }
          frame "Reinit Config" {
            n221 = Unbundle By Name(w382) -> ("Dirs.Config"=w383:path)
            n222 = call "AudioTest.Config, Deploy Config Files.vi"("SkipIfExists(F)/Overwrite(T)"=TRUE, "Config Folder"=w383) -> ("error out"=w381:errorcluster)  [unwired: 9 in]
            n223 = call <vilib>:"Clear Errors.vi"("error in (no error)"=w381) -> ()  [unwired: 5 in, 2 out]
          }
          frame Default {
          }
        }
      }
      frame "Error", Default {
        # "Do Nothing (for now)"
        n224 = call <vilib>:"Q.Enqueue Reset.vi"("Top of Q(T)"=FALSE, "Error In"=w386, "Q In"=w387) -> ()  [unwired: 7 in, 2 out]
        "Error" <- w386
      }
      frame "Exit" {
        n225 = Generate User Event(user event=w391, event data cluster=TRUE ("event data")) -> ()  [unwired: 2 in, 2 out]
        n226 = Unbundle By Name(w403) -> ("Is Child?"=w402:bool)
        n227 = property class="App"() -> ("App.Kind"=w407:T6)  [unwired: 2 in, 2 out]
        n228 = Not(x=w402) -> (.not. x?=w401:bool)
        n229 = Unbundle By Name(w399) -> ("PlotWins"=w400:cluster{"Name":string, "vi ref":refnum<vi>}[], "PlotComp"=w395:cluster{"Name":string, "vi ref":refnum<vi>})
        n230 = Equal?(x=w407, y=T6."Run Time System" ("Application:Kind")) -> (x = y?=w405:bool)
        n231 = And(x=w401, y=w405) -> (x .and. y?=w404:bool)
        n232 = for {
          tunnel: w400 -> [w410] mode=indexing
          tunnel: [w409] -> w394
          n233 = Unbundle By Name(w410) -> ("Name"=w411:string)
          n234 = call <vilib>:"Q.Enqueue Exit.vi"("Q Name"=w411) -> ("error out"=w409:errorcluster)  [unwired: 9 in, 1 out]
        }
        n235 = Unbundle By Name(w395) -> ("Name"=w396:string)
        n236 = call <vilib>:"Q.Enqueue Exit.vi"("Q Name"=w396) -> ("error out"=w392:errorcluster)  [unwired: 9 in, 1 out]
        n237 = Merge Errors(w394, w392) -> (w393:errorcluster)
        n238 = call <vilib>:"Time.Inline Delay.vi"("error in (no error)"=w393, "Wait(ms)"=u32 50) -> ("error out"=w398:errorcluster)  [unwired: 8 in, 1 out]
        n239 = case shown="True" w404 {
          selector: w404 -> [_ w412]
          tunnel: w398 -> [_ _]
          frame False {
          }
          frame True {
            n240 = Quit LabVIEW(quit? (T)=w412) -> ()
          }
        }
      }
    }
  }
